vi "PCO_METADATA_STRUCT.vi"() -> (0 "PCO_METADATA_STRUCT":T2, 1 "PCO_METADATA_STRUCT_Raw":T1, 2 "Length":u16, 3 "Raw_Length":u16)   [LabVIEW 2019, in "SDK.lvlib" / "Structures.lvlib"]
doc: "Use this template to build a VI to use as a subVI."
uses:
  Structures.lvlib
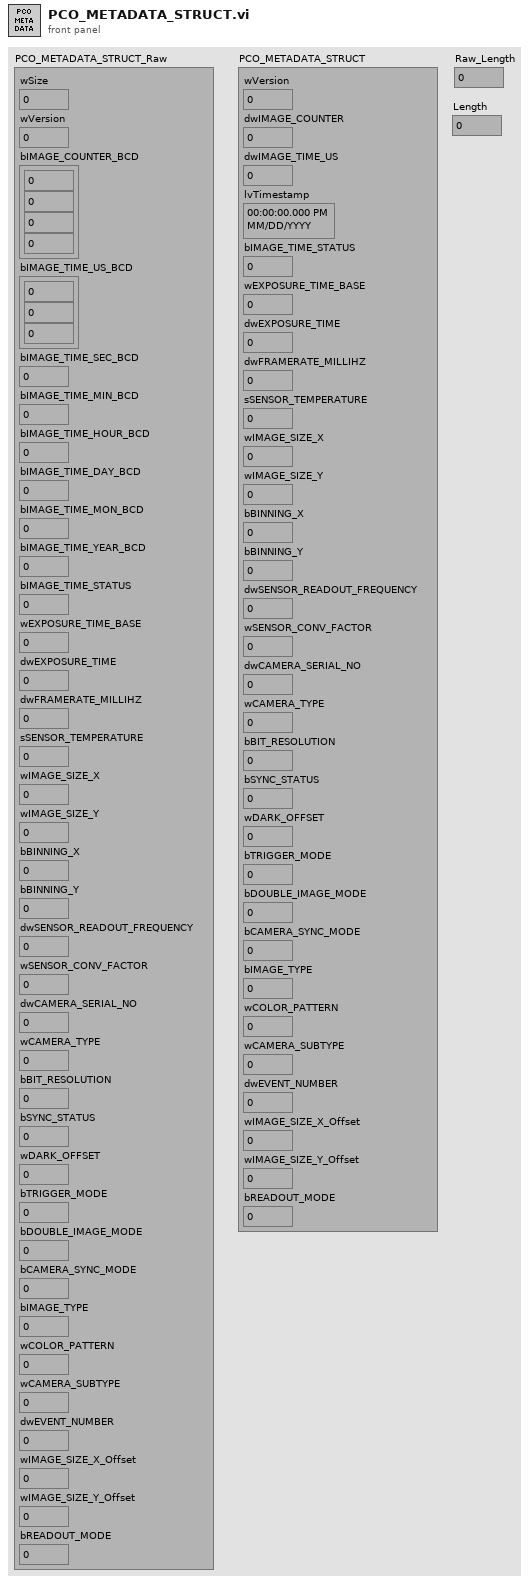
[diagram p1: front panel]
types:
  T1 = cluster{"wSize":u16, "wVersion":u16, "bIMAGE_COUNTER_BCD":cluster{u8, u8, u8, u8}, "bIMAGE_TIME_US_BCD":cluster{u8, u8, u8}, "bIMAGE_TIME_SEC_BCD":u8, "bIMAGE_TIME_MIN_BCD":u8, "bIMAGE_TIME_HOUR_BCD":u8, "bIMAGE_TIME_DAY_BCD":u8, "bIMAGE_TIME_MON_BCD":u8, "bIMAGE_TIME_YEAR_BCD":u8, "bIMAGE_TIME_STATUS":u8, "wEXPOSURE_TIME_BASE":u16, "dwEXPOSURE_TIME":u32, "dwFRAMERATE_MILLIHZ":u32, "sSENSOR_TEMPERATURE":i16, "wIMAGE_SIZE_X":u16, "wIMAGE_SIZE_Y":u16, "bBINNING_X":u8, "bBINNING_Y":u8, "dwSENSOR_READOUT_FREQUENCY":u32, "wSENSOR_CONV_FACTOR":u16, "dwCAMERA_SERIAL_NO":u32, "wCAMERA_TYPE":u16, "bBIT_RESOLUTION":u8, "bSYNC_STATUS":u8, "wDARK_OFFSET":u16, "bTRIGGER_MODE":u8, "bDOUBLE_IMAGE_MODE":u8, "bCAMERA_SYNC_MODE":u8, "bIMAGE_TYPE":u8, "wCOLOR_PATTERN":u16, "wCAMERA_SUBTYPE":u16, "dwEVENT_NUMBER":u32, "wIMAGE_SIZE_X_Offset":u16, "wIMAGE_SIZE_Y_Offset":u16, "bREADOUT_MODE":u8}
  T2 = cluster{"wVersion":u16, "dwIMAGE_COUNTER":u32, "dwIMAGE_TIME_US":u32, "lvTimestamp":timestamp, "bIMAGE_TIME_STATUS":u8, "wEXPOSURE_TIME_BASE":u16, "dwEXPOSURE_TIME":u32, "dwFRAMERATE_MILLIHZ":u32, "sSENSOR_TEMPERATURE":i16, "wIMAGE_SIZE_X":u16, "wIMAGE_SIZE_Y":u16, "bBINNING_X":u8, "bBINNING_Y":u8, "dwSENSOR_READOUT_FREQUENCY":u32, "wSENSOR_CONV_FACTOR":u16, "dwCAMERA_SERIAL_NO":u32, "wCAMERA_TYPE":u16, "bBIT_RESOLUTION":u8, "bSYNC_STATUS":u8, "wDARK_OFFSET":u16, "bTRIGGER_MODE":u8, "bDOUBLE_IMAGE_MODE":u8, "bCAMERA_SYNC_MODE":u8, "bIMAGE_TYPE":u8, "wCOLOR_PATTERN":u16, "wCAMERA_SUBTYPE":u16, "dwEVENT_NUMBER":u32, "wIMAGE_SIZE_X_Offset":u16, "wIMAGE_SIZE_Y_Offset":u16, "bREADOUT_MODE":u8}
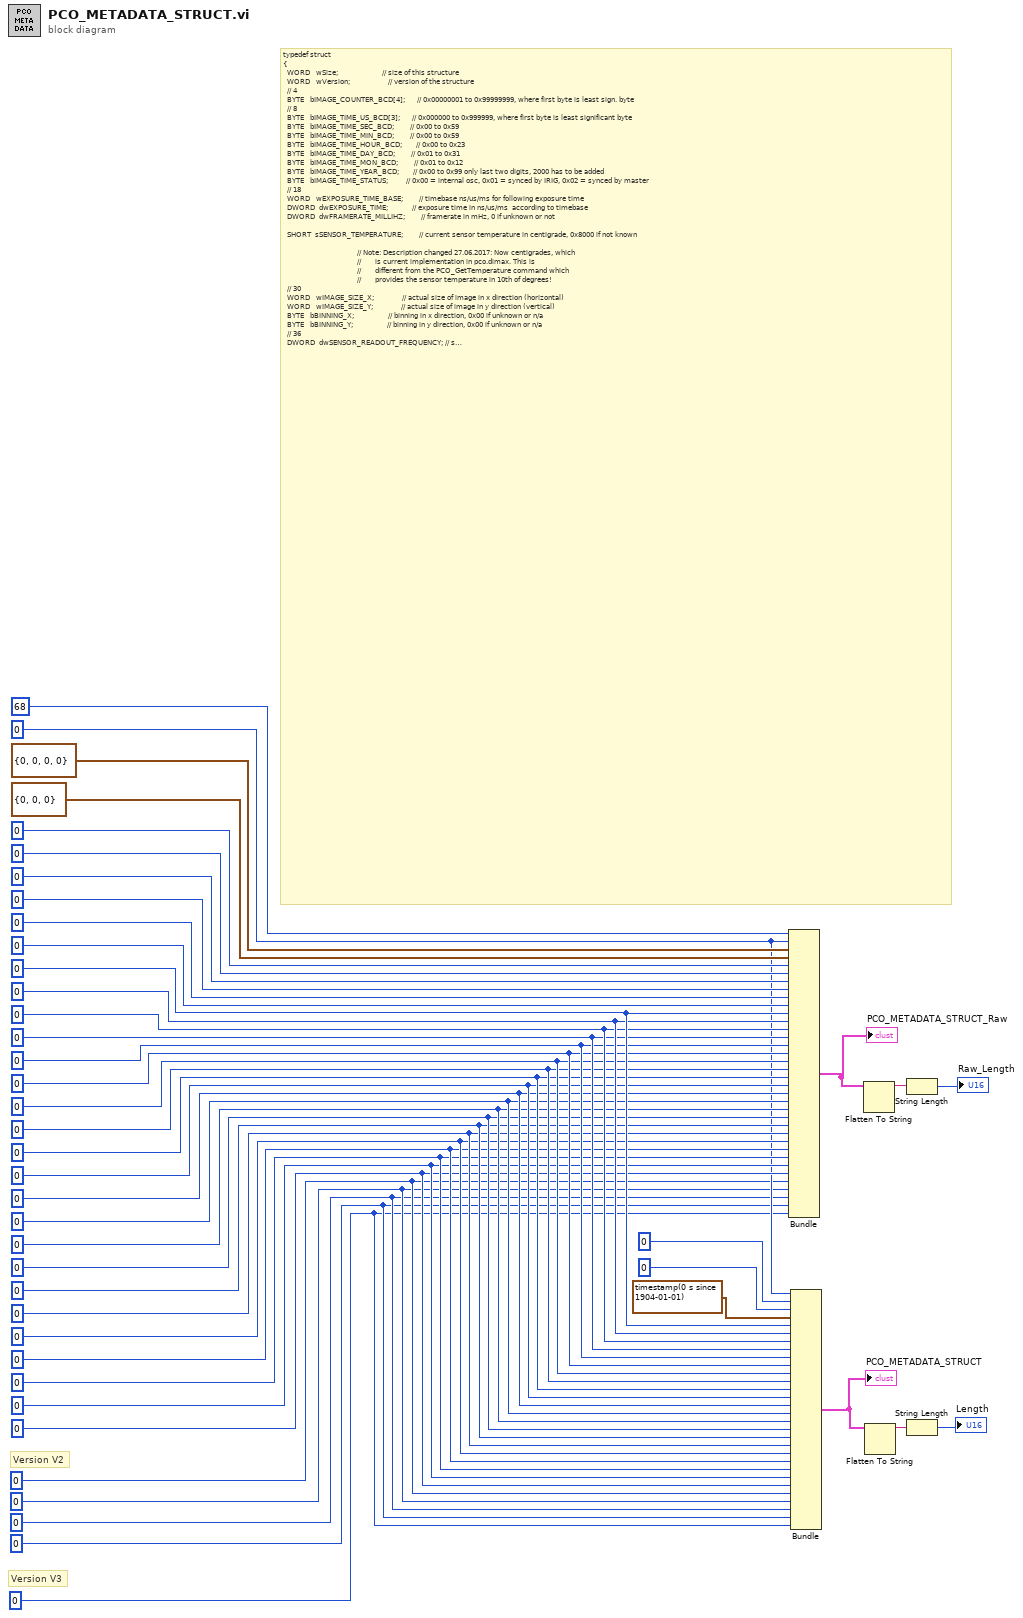
[diagram p0: block diagram]
diagram:
  w1 = u8 0 ("bREADOUT_MODE")
  w2 = u16 0 ("wIMAGE_SIZE_Y_Offset")
  w3 = u16 0 ("wIMAGE_SIZE_X_Offset")
  w4 = u32 0 ("dwEVENT_NUMBER")
  w5 = u16 0 ("wCAMERA_SUBTYPE")
  w8 = u16 0 ("wCOLOR_PATTERN")
  w9 = u8 0 ("bIMAGE_TYPE")
  w10 = u8 0 ("bCAMERA_SYNC_MODE")
  w11 = u8 0 ("bDOUBLE_IMAGE_MODE")
  w12 = u8 0 ("bTRIGGER_MODE")
  w13 = u16 0 ("wDARK_OFFSET")
  w14 = u8 0 ("bSYNC_STATUS")
  w15 = u8 0 ("bBIT_RESOLUTION")
  w16 = u16 0 ("wCAMERA_TYPE")
  w17 = u32 0 ("dwCAMERA_SERIAL_NO")
  w18 = u16 0 ("wSENSOR_CONV_FACTOR")
  w19 = u32 0 ("dwSENSOR_READOUT_FREQUENCY")
  w20 = u8 0 ("bBINNING_Y")
  w21 = u8 0 ("bBINNING_X")
  w22 = u16 0 ("wIMAGE_SIZE_Y")
  w23 = u16 0 ("wIMAGE_SIZE_X")
  w24 = i16 0 ("sSENSOR_TEMPERATURE")
  w25 = u32 0 ("dwFRAMERATE_MILLIHZ")
  w26 = u32 0 ("dwEXPOSURE_TIME")
  w27 = u16 0 ("wEXPOSURE_TIME_BASE")
  w28 = u8 0 ("bIMAGE_TIME_STATUS")
  w7 = u16 0 ("wVersion")
  # "Version V3"
  # "Version V2"
  # "typedef struct\n{\n  WORD   wSize;                      // size of this structure\n  WORD   wVersion;                   // version of the structure\n  // 4\n  BYTE   bIMAGE_COUNTER_BCD[4];      // 0x00000001 to 0x99999999, where first byte is least sign. byte\n  // 8\n  BYTE   bIMAGE_TIME_US_BCD[3];      // 0x000000 to 0x999999, where first byte is least significant byte\n  BYTE   bIMAGE_TIME_SEC_BCD;        // 0x00 to 0x59\n  BYTE   bIMAGE_TIME_MIN_BCD;        // 0x00 to 0x59\n  BYTE   bIMAGE_TIME_HOUR_BCD;       // 0x00 to 0x23\n  BYTE   bIMAGE_TIME_DAY_BCD;        // 0x01 to 0x31\n  BYTE   bIMAGE_TIME_MON_BCD;        // 0x01 to 0x12\n  BYTE   bIMAGE_TIME_YEAR_BCD;       // 0x00 to 0x99 only last two digits, 2000 has to be added\n  BYTE   bIMAGE_TIME_STATUS;         // 0x00 = internal osc, 0x01 = synced by IRIG, 0x02 = synced by master\n  // 18\n  WORD   wEXPOSURE_TIME_BASE;        // timebase ns/us/ms for following exposure time\n  DWORD  dwEXPOSURE_TIME;            // exposure time in ns/us/ms  according to timebase\n  DWORD  dwFRAMERATE_MILLIHZ;        // framerate in mHz, 0 if unknown or not\n\n  SHORT  sSENSOR_TEMPERATURE;        // current sensor temperature in centigrade, 0x8000 if not known\n\n                                     // Note: Description changed 27.06.2017: Now centigrades, which\n                                     //       is current implementation in pco.dimax. This is \n                                     //       different from the PCO_GetTemperature command which\n                                     //       provides the sensor temperature in 10th of degrees!\n  // 30\n  WORD   wIMAGE_SIZE_X;              // actual size of image in x direction (horizontal)\n  WORD   wIMAGE_SIZE_Y;              // actual size of image in y direction (vertical)\n  BYTE   bBINNING_X;                 // binning in x direction, 0x00 if unknown or n/a\n  BYTE   bBINNING_Y;                 // binning in y direction, 0x00 if unknown or n/a\n  // 36\n  DWORD  dwSENSOR_READOUT_FREQUENCY; // sensor readout frequency in Hz, 0 if unknown\n  WORD   wSENSOR_CONV_FACTOR;        // sensor conversions factor in e-/ct, 0 if unknown\n  // 42\n  DWORD  dwCAMERA_SERIAL_NO;         // camera serial no, 0 if unknown\n  WORD   wCAMERA_TYPE;               // type of pco camera taking the images, see SDK, 0 if unknown\n  BYTE   bBIT_RESOLUTION;            // number of valid bits of the pixel values, e.g. 12 for the pco.dimax\n  BYTE   bSYNC_STATUS;               // status of PLL for external synchronisation (100 Hz or 1 kHz): 0 = off, 1 = locked\n  WORD   wDARK_OFFSET;               // nominal dark offset in counts, 0xFFFF if unknown, current dark offset may differ\n  // 52\n  BYTE   bTRIGGER_MODE;              // exposure trigger mode, see PCO SDK\n  BYTE   bDOUBLE_IMAGE_MODE;         // 0x00 = standard, 0x01 = double image (PIV) mode\n  BYTE   bCAMERA_SYNC_MODE;          // see PCO SDK\n  BYTE   bIMAGE_TYPE;                // 0x01 ist b/w, 0x02 is color bayer pattern, 0x10 is RGB mode\n  WORD   wCOLOR_PATTERN;             // bayer pattern color mask, same as for SDK command \"Get Camera Description\", 0 if n/a\n  // 58 - structure V2 starting here\n  WORD   wCAMERA_SUBTYPE;            // sub-type of pco camera taking the images, see SDK, 0 if unknown\n  DWORD  dwEVENT_NUMBER;             // application dependent event number\n  // 64 bytes ..\n  WORD   wIMAGE_SIZE_X_Offset;       // actual x offset in case of ROI (X0) in x direction (horizontal)\n  WORD   wIMAGE_SIZE_Y_Offset;       // actual y offset in case of ROI (Y0) in y direction (vertical)\n  // 68 bytes - structure V3 starting here\n  BYTE      bREADOUT_MODE;              //  [7]: readout direction: 0 = normal, 1 = reverse; [6:0]:: readout mode\n  // 69 bytes..\n}\nPCO_METADATA_STRUCT;"
  n1 = Bundle("wSize"=u16 68, "wVersion"=w7, "bIMAGE_COUNTER_BCD"=cluster{u8, u8, u8, u8} {0, 0, 0, 0}, "bIMAGE_TIME_US_BCD"=cluster{u8, u8, u8} {0, 0, 0}, "bIMAGE_TIME_SEC_BCD"=u8 0, "bIMAGE_TIME_MIN_BCD"=u8 0, "bIMAGE_TIME_HOUR_BCD"=u8 0, "bIMAGE_TIME_DAY_BCD"=u8 0, "bIMAGE_TIME_MON_BCD"=u8 0, "bIMAGE_TIME_YEAR_BCD"=u8 0, "bIMAGE_TIME_STATUS"=w28, "wEXPOSURE_TIME_BASE"=w27, "dwEXPOSURE_TIME"=w26, "dwFRAMERATE_MILLIHZ"=w25, "sSENSOR_TEMPERATURE"=w24, "wIMAGE_SIZE_X"=w23, "wIMAGE_SIZE_Y"=w22, "bBINNING_X"=w21, "bBINNING_Y"=w20, "dwSENSOR_READOUT_FREQUENCY"=w19, "wSENSOR_CONV_FACTOR"=w18, "dwCAMERA_SERIAL_NO"=w17, "wCAMERA_TYPE"=w16, "bBIT_RESOLUTION"=w15, "bSYNC_STATUS"=w14, "wDARK_OFFSET"=w13, "bTRIGGER_MODE"=w12, "bDOUBLE_IMAGE_MODE"=w11, "bCAMERA_SYNC_MODE"=w10, "bIMAGE_TYPE"=w9, "wCOLOR_PATTERN"=w8, "wCAMERA_SUBTYPE"=w5, "dwEVENT_NUMBER"=w4, "wIMAGE_SIZE_X_Offset"=w3, "wIMAGE_SIZE_Y_Offset"=w2, "bREADOUT_MODE"=w1) -> (w40:T1)  [unwired: 1 in]
  "PCO_METADATA_STRUCT_Raw" <- w40
  n2 = Bundle("wVersion"=w7, "dwIMAGE_COUNTER"=u32 0, "dwIMAGE_TIME_US"=u32 0, "lvTimestamp"=timestamp(0 s since 1904-01-01), "bIMAGE_TIME_STATUS"=w28, "wEXPOSURE_TIME_BASE"=w27, "dwEXPOSURE_TIME"=w26, "dwFRAMERATE_MILLIHZ"=w25, "sSENSOR_TEMPERATURE"=w24, "wIMAGE_SIZE_X"=w23, "wIMAGE_SIZE_Y"=w22, "bBINNING_X"=w21, "bBINNING_Y"=w20, "dwSENSOR_READOUT_FREQUENCY"=w19, "wSENSOR_CONV_FACTOR"=w18, "dwCAMERA_SERIAL_NO"=w17, "wCAMERA_TYPE"=w16, "bBIT_RESOLUTION"=w15, "bSYNC_STATUS"=w14, "wDARK_OFFSET"=w13, "bTRIGGER_MODE"=w12, "bDOUBLE_IMAGE_MODE"=w11, "bCAMERA_SYNC_MODE"=w10, "bIMAGE_TYPE"=w9, "wCOLOR_PATTERN"=w8, "wCAMERA_SUBTYPE"=w5, "dwEVENT_NUMBER"=w4, "wIMAGE_SIZE_X_Offset"=w3, "wIMAGE_SIZE_Y_Offset"=w2, "bREADOUT_MODE"=w1) -> (w39:T2)  [unwired: 1 in]
  "PCO_METADATA_STRUCT" <- w39
  n3 = Flatten To String(anything=w40) -> (data string=w44:string)  [unwired: 3 in, 2 out]
  n4 = Flatten To String(anything=w39) -> (data string=w45:string)  [unwired: 3 in, 2 out]
  n5 = String Length(string=w44) -> (length=→"Raw_Length":i32)
  n6 = String Length(string=w45) -> (length=→"Length":i32)
